vi "Measurements Scan.vi"(8 "error in (no error)":errorcluster, 11 "TestStand Controller in":refnum<class "Controller API.lvclass">) -> (0 "error out":errorcluster, 3 "TestStand Controller out":refnum<class "Controller API.lvclass">)   [LabVIEW 2016, in "Controller API.lvlib" / "Controller API.lvclass"]
uses:
  <userlib>/Measurement Utility API/Controller API.lvclass
  C:/Program Files (x86)/National Instruments/LabVIEW 2016/user.lib/Common Components/Controller/Controller.lvclass
  <userlib>/Common Components/Controller/Controller.lvclass/Controller.ctl
  <userlib>/Common Components/Controller/Accessors/Read Root Path.vi
  <userlib>/Common Components/Controller/Controller.lvclass
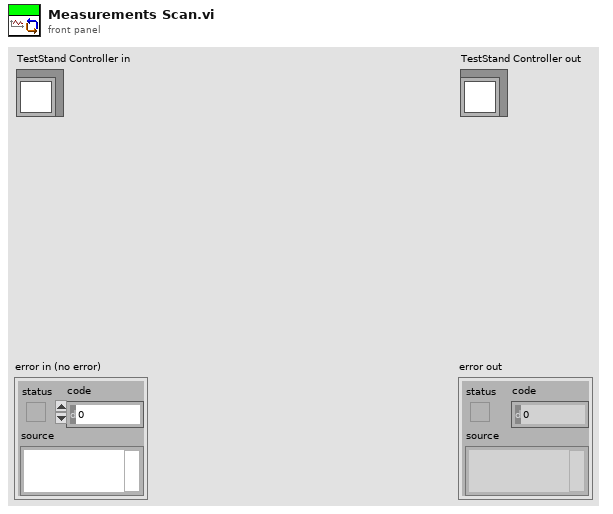
[diagram p1: front panel]
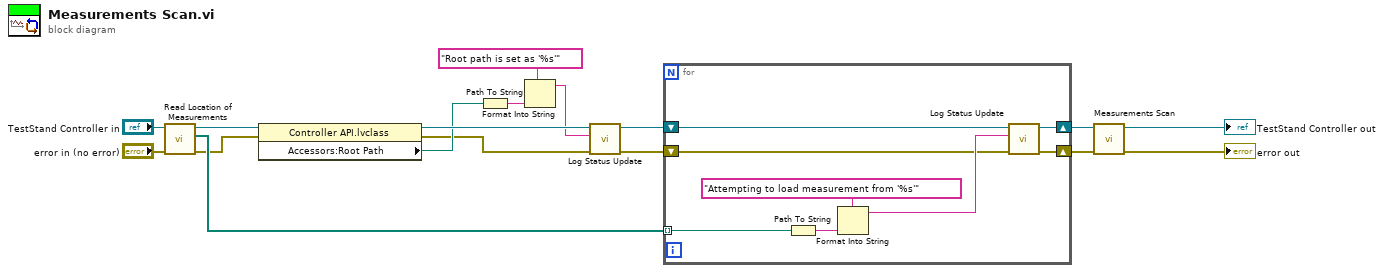
[diagram p0: block diagram]
diagram:
  n1 = call <userlib>:"Read Location of Measurements.vi"("error in (no error)"="error in (no error)", "Controller in"="TestStand Controller in") -> ("error out"=w4:errorcluster, "Array of Measurement Location"=w13:path[], "Controller out"=w12:refnum<class "Controller API.lvclass">)  [unwired: 7 in]
  n2 = property class="Controller API.lvclass"(reference=w12, error in=w4) -> (reference out=w9:refnum<class "Controller API.lvclass">, error out=w3:errorcluster, "Accessors:Root Path"=w8:path)
  n3 = Path To String(path=w8) -> (string=w6:string)
  n4 = Format Into String(format string="Root path is set as '%s'", w6) -> (resulting string=w5:string)  [unwired: 2 in, 1 out]
  n5 = call-dynamic "Log Status Update.vi"("error in (no error)"=w3, "String"=w5, "TestStand Controller in"=w9) -> ("error out"=w2:errorcluster, "TestStand Controller out"=w10:refnum<class "Controller API.lvclass">)  [unwired: 7 in]
  n6 = for {
    tunnel: w13 -> [w25] mode=indexing
    shift-right: [w23] -> w11
    shift-left: w10 -> [w24]
    shift-right: [w18] -> w1
    shift-left: w2 -> [w19]
    n7 = Path To String(path=w25) -> (string=w21:string)
    n8 = Format Into String(format string="Attempting to load measurement from '%s'", w21) -> (resulting string=w22:string)  [unwired: 2 in, 1 out]
    n9 = call-dynamic "Log Status Update.vi"("error in (no error)"=w19, "String"=w22, "TestStand Controller in"=w24) -> ("error out"=w18:errorcluster, "TestStand Controller out"=w23:refnum<class "Controller API.lvclass">)  [unwired: 7 in]
  }
  n10 = call-parent "Measurements Scan.vi"("error in (no error)"=w1, "Controller in"=w11) -> ("error out"=→"error out":errorcluster, "Controller out"=→"TestStand Controller out":refnum<class "Controller API.lvclass">)  [unwired: 8 in]
